vi "Convert AI Robot to Robot Command.vi"(1 "Input Array":T2[](array[typedef])) -> (0 "Output Array":T1[](array[typedef]))   [LabVIEW 2016]
uses:
  AI Robot.ctl
  grSim/grSim Robot Command.ctl
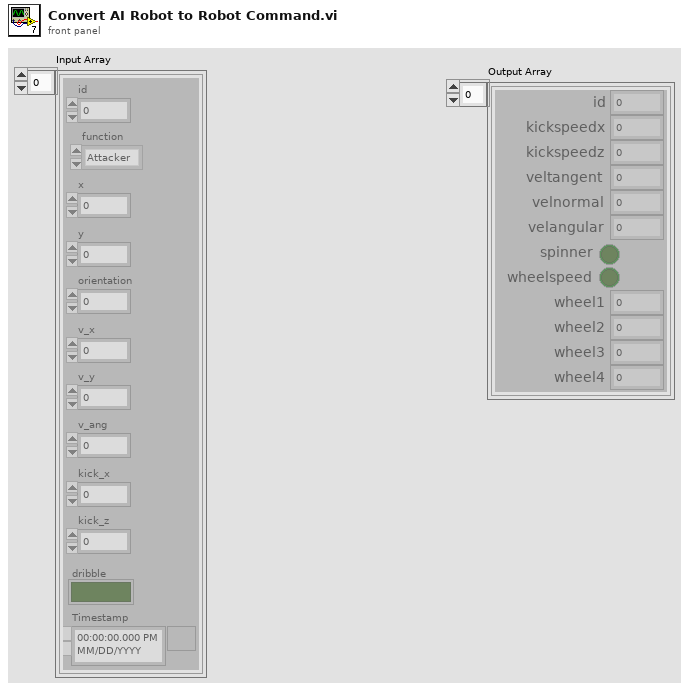
[diagram p1: front panel]
types:
  T1 = typedef "grSim Robot Command.ctl" = cluster{"id":u32, "kickspeedx":sgl, "kickspeedz":sgl, "veltangent":sgl, "velnormal":sgl, "velangular":sgl, "spinner":bool, "wheelspeed":bool, "wheel1":sgl, "wheel2":sgl, "wheel3":sgl, "wheel4":sgl}
  T2 = typedef "AI Robot.ctl" = cluster{"id":u32, "function":enum16{"Attacker", "Goalie", "Defender"}, "x":dbl, "y":dbl, "orientation":dbl, "v_x":dbl, "v_y":dbl, "v_ang":dbl, "kick_x":dbl, "kick_z":dbl, "dribble":bool, "Timestamp":timestamp}
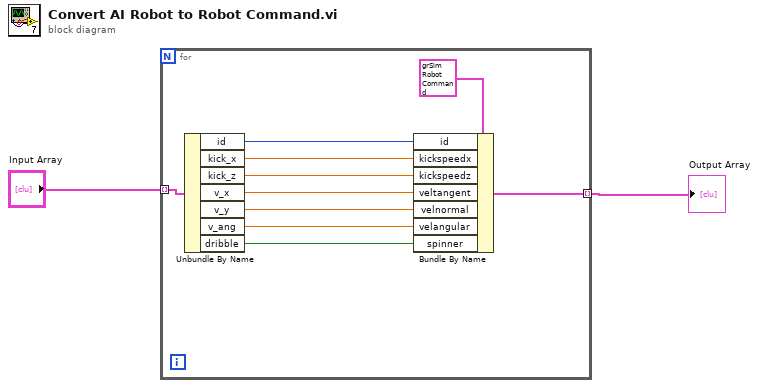
[diagram p0: block diagram]
diagram:
  n1 = for {
    tunnel: "Input Array" -> [w12] mode=indexing
    tunnel: [w3] -> w1 mode=indexing
    n2 = Unbundle By Name(w12) -> ("id"=w10:u32, "kick_x"=w9:dbl, "kick_z"=w8:dbl, "v_x"=w7:dbl, "v_y"=w6:dbl, "v_ang"=w5:dbl, "dribble"=w4:bool)
    n3 = Bundle By Name(cluster=T1 {"id"=0, "kickspeedx"=0.0, "kickspeedz"=0.0, "veltangent"=0.0, "velnormal"=0.0, "velangular"=0.0, "spinner"=FALSE, "wheelspeed"=FALSE, "wheel1"=0.0, "wheel2"=0.0, "wheel3"=0.0, "wheel4"=0.0} ("grSim Robot Command"), "id"=w10, "kickspeedx"=w9, "kickspeedz"=w8, "veltangent"=w7, "velnormal"=w6, "velangular"=w5, "spinner"=w4) -> (w3:T1)
  }
  "Output Array" <- w1
